vi "Parse RSB Host Telemetry.vi"(10 "Variant":variant) -> (2 "Telemetry_Data":T1 {"Timing" format="%#_6p"; "Data" format="%04x"})   [LabVIEW 2019]
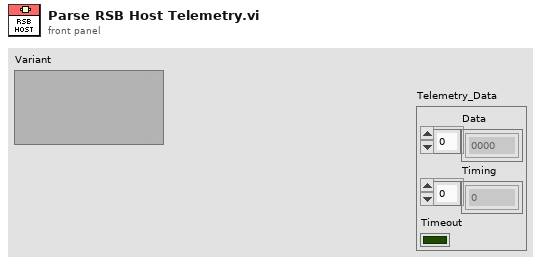
[diagram p1: front panel]
types:
  T1 = cluster{"Data":u16[], "Timing":dbl[], "Timeout":bool}
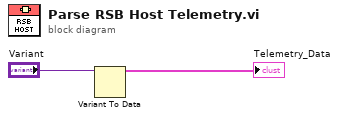
[diagram p0: block diagram]
diagram:
  n1 = Variant To Data(Variant="Variant") -> (data=→"Telemetry_Data":T1)  [unwired: 2 in, 1 out]
